vi "ChangeEpsilon.vi"(10 "new epsilon":dbl, 11 "RVCLibrary_Bug2 in":refnum<class "RVCLibrary_Bug2.lvclass">) -> (3 "RVCLibrary_Bug2 out":refnum<class "RVCLibrary_Bug2.lvclass">)   [LabVIEW 2013, in "RVCLibrary_Bug2.lvclass"]
uses:
  RVCLibrary_Bug2.lvclass
  RVCLibrary_Bug2.lvclass/RVCLibrary_Bug2.ctl
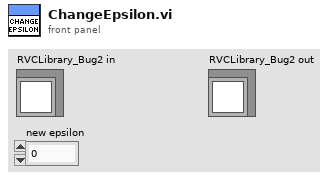
[diagram p1: front panel]
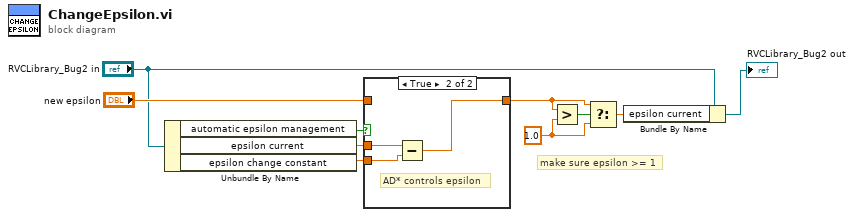
[diagram p0: block diagram]
diagram:
  w9 = 1.0 ("y")
  # "make sure epsilon >= 1"
  n1 = Unbundle By Name("RVCLibrary_Bug2 in") -> ("automatic epsilon management"=w7:bool, "epsilon current"=w6:dbl, "epsilon change constant"=w4:dbl)
  n2 = case shown="True" w7 {
    tunnel: [w11 w12] -> w8
    tunnel: w6 -> [_ w13]
    tunnel: "new epsilon" -> [w11 _]
    tunnel: w4 -> [_ w14]
    frame False {
    }
    frame True {
      # "AD* controls epsilon"
      n3 = Subtract(x=w13, y=w14) -> (x-y=w12:dbl)
    }
  }
  n4 = Greater?(x=w8, y=w9) -> (0:w10:bool)
  n5 = Select(t=w8, s=w10, f=w9) -> (s? t:f=w3:dbl)
  n6 = Bundle By Name(cluster="RVCLibrary_Bug2 in", "epsilon current"=w3) -> (→"RVCLibrary_Bug2 out":refnum<class "RVCLibrary_Bug2.lvclass">)
